vi "Table, Append Row Number.vi"(8 "error in":errorcluster, 11 "Tbl Refnum":refnum<vi>) -> (0 "error out":errorcluster, 3 "Tbl Refnum out":refnum<vi>)   [LabVIEW 2010]
doc: "This function appends the row number onto the row header vector string."
panel:
  out "row index":i32
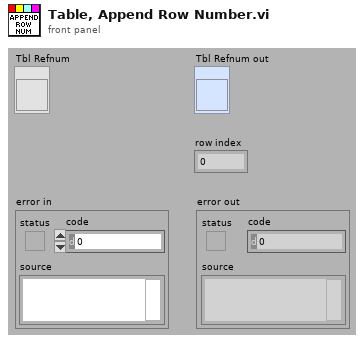
[diagram p1: front panel]
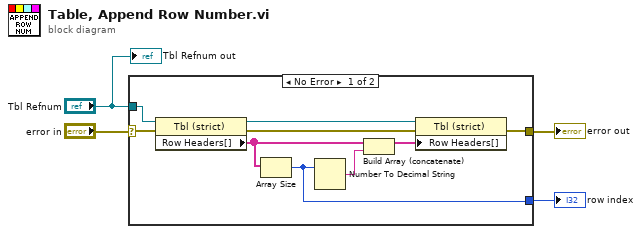
[diagram p0: block diagram]
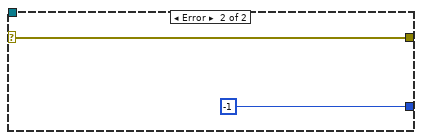
[diagram p2: hidden frame]
diagram:
  n1 = case shown="No Error" "error in" {
    selector: "error in" -> [w8 w15]
    tunnel: "Tbl Refnum" -> [w7 _]
    tunnel: [w11 w15] -> w3
    tunnel: [w5 -1] -> w1
    frame No Error {
      n2 = property class="Tbl (strict)"(reference=w7, error in=w8) -> (reference out=w13:refnum<vi>, error out=w12:errorcluster, "Row Headers[]"=w6:string[])
      n3 = Array Size(array=w6) -> (size(s)=w5:i32)
      n4 = Number To Decimal String(number=w5) -> (decimal integer string=w9:string)  [unwired: 1 in]
      n5 = Build Array (concatenate)(w6, w9) -> (w10:string[])
      n6 = property class="Tbl (strict)"(reference=w13, error in=w12, "Row Headers[]"=w10) -> (error out=w11:errorcluster)  [unwired: 1 out]
    }
    frame Error {
    }
  }
  "error out" <- w3
  "row index" <- w1
  "Tbl Refnum out" <- "Tbl Refnum"
